vi "设置UI.vi"(11 "站点":string) -> ()   [LabVIEW 2016]
uses:
  <vilib>/Utility/config.llb/NI_LVConfig.lvlib
panel:
  in  "关闭":bool
  in  "启用":bool
  out "内容":string
  in  "测试":bool
  out "error out":errorcluster caption="错误输出"
  out "body":string caption="体部"
  out "headers":string caption="头部"
  in  "PhoneNumbers":string
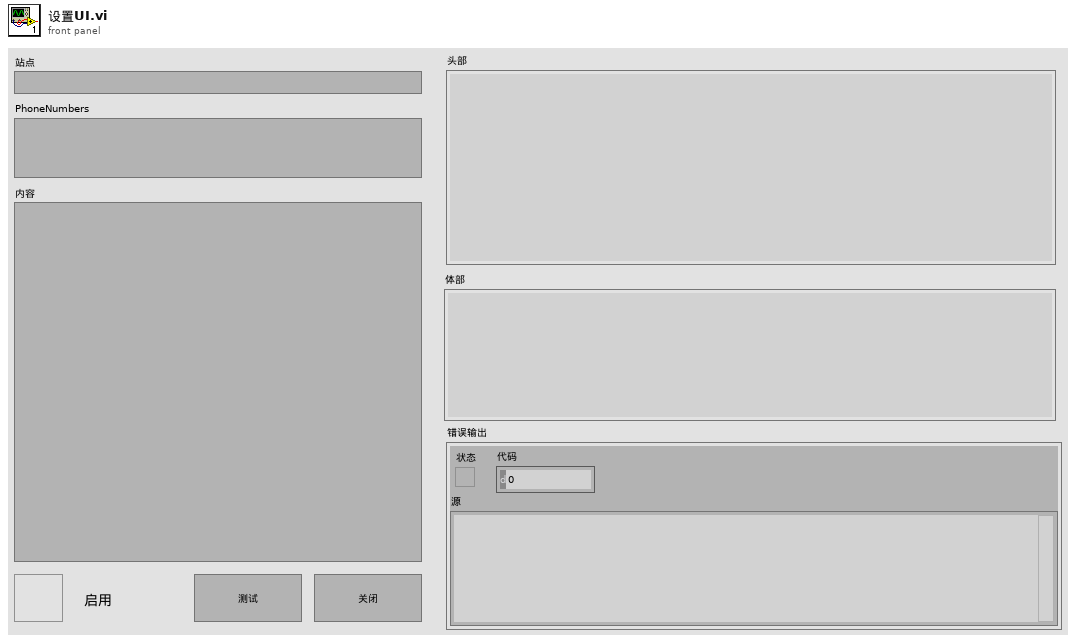
[diagram p1: front panel]
types:
  T1 = typedef "NI_LVConfig.lvlib/Config Data RefNum.ctl" = refnum<k1>
  T2 = enum32{"Invalid", "Standard", "Closed", "Hidden", "Minimized", "Maximized"}
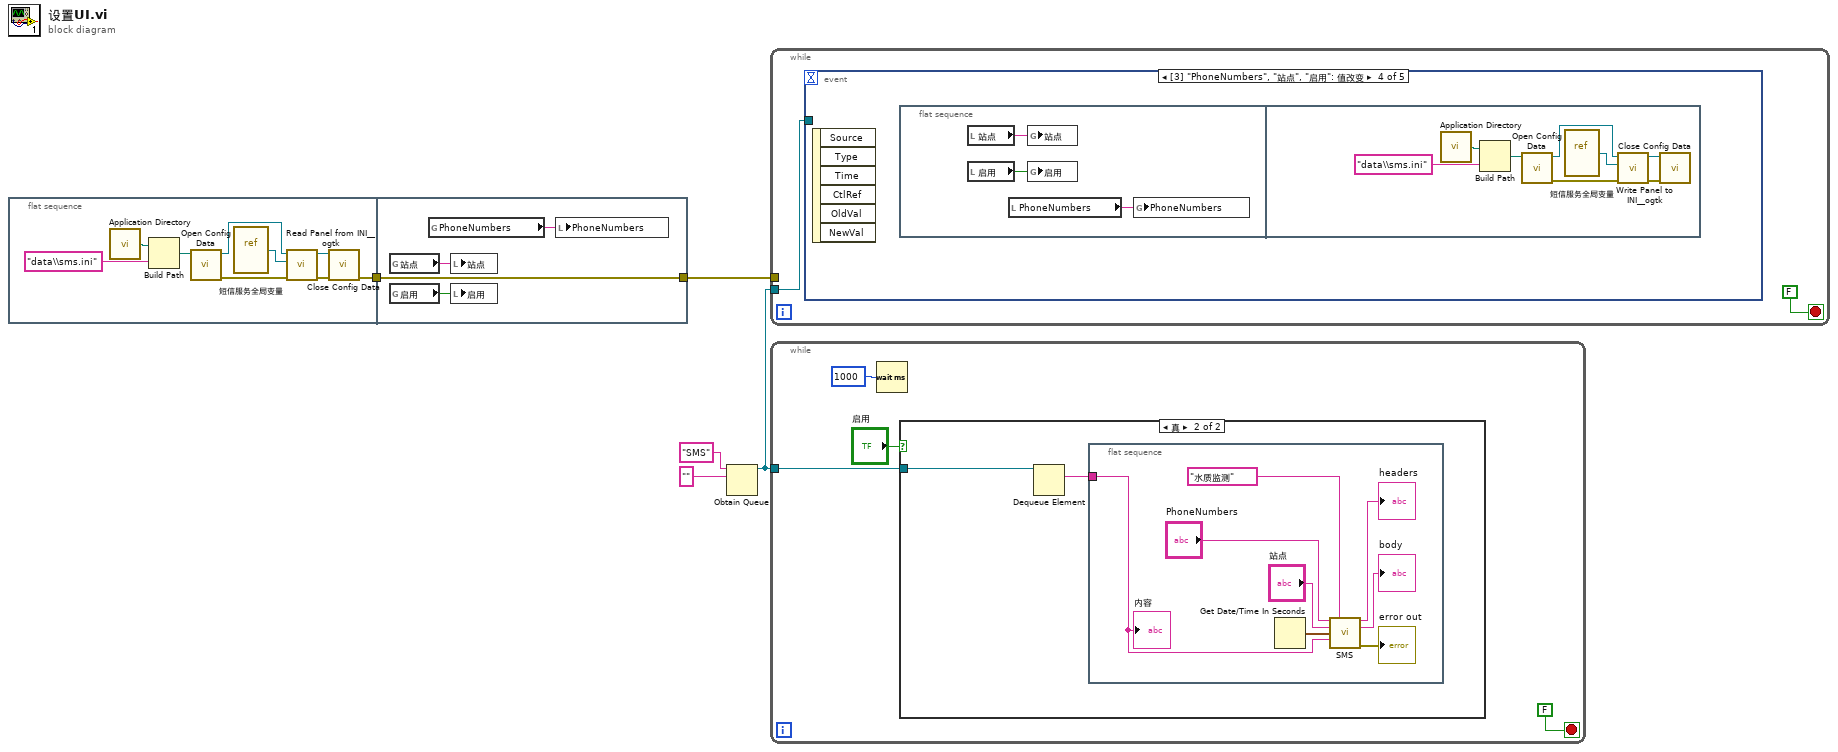
[diagram p0: block diagram]
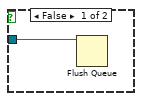
[diagram p2: hidden frame]
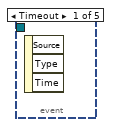
[diagram p3: hidden frame]
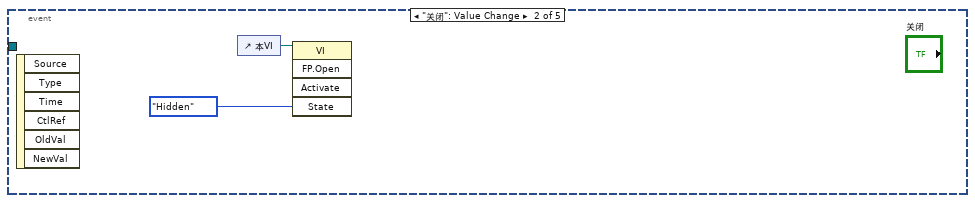
[diagram p4: hidden frame]
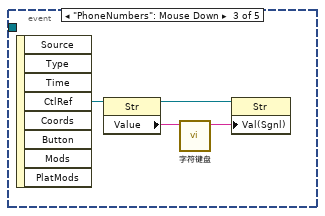
[diagram p5: hidden frame]
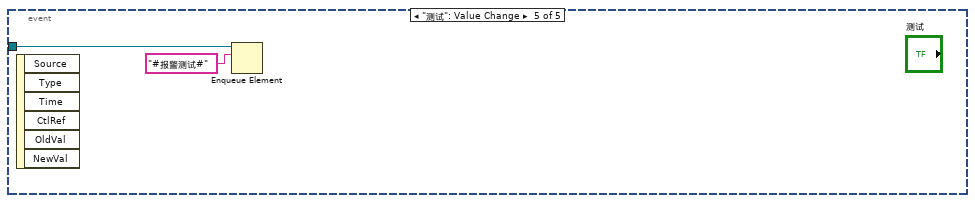
[diagram p6: hidden frame]
diagram:
  n1 = flat-sequence {
    tunnel: [w6] -> w4
    tunnel: [w18] -> w5
    tunnel: w4 -> [w18]
    frame #0 {
      n2 = call <vilib>:"Application Directory.vi"() -> ("Application Directory"=w12:path)
      n3 = Build Path(base path=w12, name or relative path="data\\sms.ini" ("名称或相对路径")) -> (appended path=w13:path)
      n4 = call <vilib>:"Open Config Data.vi"("configuration file path"=w13) -> ("error out"=w8:errorcluster, "refnum"=w7:T1)  [unwired: 8 in, 1 out]
      n5 = vi-ref "短信服务全局变量.vi"() -> (w11:refnum<vi>)
      n6 = call <userlib>:"Read Panel from INI__ogtk.vi"("error in (no error)"=w8, "VI ref"=w11, "refnum"=w7) -> ("error out"=w10:errorcluster, "refnum out"=w9:T1)  [unwired: 7 in]
      n7 = call <vilib>:"Close Config Data.vi"("error in (no error)"=w10, "refnum"=w9) -> ("error out"=w6:errorcluster)  [unwired: 8 in, 1 out]
    }
    frame #1 {
      n8 = global read "短信服务全局变量.vi" "站点"() -> (w16:string)
      n9 = global read "短信服务全局变量.vi" "启用"() -> (w15:bool)
      n10 = global read "短信服务全局变量.vi" "PhoneNumbers"() -> (w17:string)
      n11 = local write "站点"(w16) -> ()
      n12 = local write "启用"(w15) -> ()
      n13 = local write "PhoneNumbers"(w17) -> ()
    }
  }
  n14 = Obtain Queue(name (unnamed)="SMS" ("名称（未命名）"), element data type="" ("名称（未命名）")) -> (queue out=w1:refnum<queue>)  [unwired: 3 in, 2 out]
  n15 = while {
    tunnel: w5 -> [_]
    tunnel: w1 -> [w19]
    stop <- FALSE stop-if-true
    n16 = event shown="[3] \"PhoneNumbers\", \"站点\", \"启用\": 值改变" {
      selector: _ -> [_ _ _ _ _]
      dyn-events: _ -> [_ _ _ _ _]
      timeout: _ -> [_ _ _ _ _]
      tunnel: w19 -> [_ _ _ _ w39]
      event Timeout {
        n17 = event-data() -> ()  [unwired: 1 in, 3 out]
      }
      event "关闭": Value Change {
        n18 = event-data() -> ()  [unwired: 1 in, 6 out]
        n19 = control-ref of="本VI"() -> (w21:refnum<vi>)
        n20 = invoke class="VI" method="FP.Open"(reference=w21, "State"=T2."Hidden" ("状态")) -> ()  [unwired: 3 in, 5 out]
      }
      event "PhoneNumbers": Mouse Down {
        n21 = event-data() -> ("CtlRef"=w26:refnum<vi>)  [unwired: 1 in, 7 out]
        n22 = property class="Str"(reference=w26) -> (reference out=w23:refnum<vi>, "Value"=w25:string)  [unwired: 1 in, 1 out]
        n23 = call "字符键盘.vi"("Old String"=w25) -> ("String"=w24:string)  [unwired: 10 in]
        n24 = property class="Str"(reference=w23, "Val(Sgnl)"=w24) -> ()  [unwired: 1 in, 2 out]
      }
      event "PhoneNumbers", "站点", "启用": Value Change {
        n25 = event-data() -> ()  [unwired: 1 in, 6 out]
        n26 = flat-sequence {
          frame #0 {
            n27 = local read "站点"() -> (w29:string)
            n28 = local read "启用"() -> (w27:bool)
            n29 = local read "PhoneNumbers"() -> (w28:string)
            n30 = global write "短信服务全局变量.vi" "站点"(w29) -> ()
            n31 = global write "短信服务全局变量.vi" "启用"(w27) -> ()
            n32 = global write "短信服务全局变量.vi" "PhoneNumbers"(w28) -> ()
          }
          frame #1 {
            n33 = call <vilib>:"Application Directory.vi"() -> ("Application Directory"=w32:path)
            n34 = Build Path(base path=w32, name or relative path="data\\sms.ini" ("名称或相对路径")) -> (appended path=w31:path)
            n35 = call <vilib>:"Open Config Data.vi"("configuration file path"=w31) -> ("error out"=w36:errorcluster, "refnum"=w37:T1)  [unwired: 8 in, 1 out]
            n36 = vi-ref "短信服务全局变量.vi"() -> (w33:refnum<vi>)
            n37 = call <userlib>:"Write Panel to INI__ogtk.vi"("error in (no error)"=w36, "VI ref"=w33, "refnum"=w37) -> ("error out"=w34:errorcluster, "refnum out"=w35:T1)  [unwired: 7 in]
            n38 = call <vilib>:"Close Config Data.vi"("error in (no error)"=w34, "refnum"=w35) -> ()  [unwired: 8 in, 2 out]
          }
        }
      }
      event "测试": Value Change {
        n39 = event-data() -> ()  [unwired: 1 in, 6 out]
        n40 = Enqueue Element(queue=w39, element="#报警测试#" ("内容")) -> ()  [unwired: 2 in, 3 out]
      }
    }
  }
  n41 = while {
    tunnel: w1 -> [w41]
    stop <- FALSE stop-if-true
    n42 = Wait (ms)(milliseconds to wait=u32 1000 ("等待时间（毫秒）")) -> ()  [unwired: 1 out]
    n43 = case shown="真" "启用" {
      tunnel: w41 -> [w44 w46]
      frame False {
        n44 = Flush Queue(queue=w44) -> ()  [unwired: 1 in, 3 out]
      }
      frame True {
        n45 = Dequeue Element(queue=w46) -> (element=w45:string)  [unwired: 2 in, 3 out]
        n46 = flat-sequence {
          tunnel: w45 -> [w54]
          frame #0 {
            n47 = Get Date/Time In Seconds() -> (seconds since 1Jan1904=w51:timestamp)
            n48 = call "SMS.vi"("PhoneNumbers"="PhoneNumbers", "SignName"="水质监测", "站点"="站点", "时间标识"=w51, "内容"=w54) -> ("headers"=→"headers":string, "body"=→"body":string, "error out"=→"error out":errorcluster)  [unwired: 8 in]
            "内容" <- w54
          }
        }
      }
    }
  }
